vi "Request Refnum Release.vi"(8 "error in":errorcluster) -> (0 "error out":errorcluster)   [LabVIEW 2020, in "SECS Scenarios.lvlib" / "Scenarios Class.lvclass"]
uses:
  Scenarios Class.lvclass
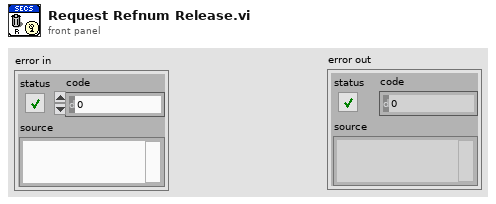
[diagram p1: front panel]
types:
  T1 = typedef "SECS Scenarios.lvlib/Scenarios Class.lvclass/Request Refnum.ctl" = cluster{"11-Alarm Management":refnum<user-event>, "07-Event Report From Equipment":refnum<user-event>, "14-Process Program Creating Editing or Deleting":refnum<user-event>, "21-Material Movement":refnum<user-event>, "23-Equipment Sends Information to Host":refnum<user-event>, "24-Host Accepts On-Line Request from Equipment":refnum<user-event>, "25-Host Refuses On-Line Request":refnum<user-event>, "29-Equipment Requests Time Value from Host":refnum<user-event>, "33-Update Trace Data":refnum<user-event>}
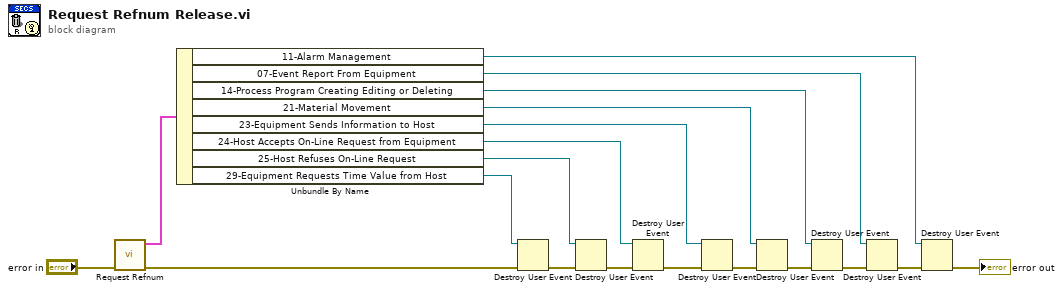
[diagram p0: block diagram]
diagram:
  n1 = call "Request Refnum.vi"("error in"="error in") -> ("error out"=w1:errorcluster, "Request Refnum"=w17:T1)  [unwired: 9 in]
  n2 = Unbundle By Name(w17) -> ("11-Alarm Management"=w8:refnum<user-event>, "07-Event Report From Equipment"=w9:refnum<user-event>, "14-Process Program Creating Editing or Deleting"=w10:refnum<user-event>, "21-Material Movement"=w11:refnum<user-event>, "23-Equipment Sends Information to Host"=w12:refnum<user-event>, "24-Host Accepts On-Line Request from Equipment"=w7:refnum<user-event>, "25-Host Refuses On-Line Request"=w4:refnum<user-event>, "29-Equipment Requests Time Value from Host"=w2:refnum<user-event>)
  n3 = Destroy User Event(user event=w2, error in=w1) -> (error out=w3:errorcluster)
  n4 = Destroy User Event(user event=w4, error in=w3) -> (error out=w5:errorcluster)
  n5 = Destroy User Event(user event=w7, error in=w5) -> (error out=w6:errorcluster)
  n6 = Destroy User Event(user event=w12, error in=w6) -> (error out=w15:errorcluster)
  n7 = Destroy User Event(user event=w11, error in=w15) -> (error out=w14:errorcluster)
  n8 = Destroy User Event(user event=w10, error in=w14) -> (error out=w13:errorcluster)
  n9 = Destroy User Event(user event=w9, error in=w13) -> (error out=w16:errorcluster)
  n10 = Destroy User Event(user event=w8, error in=w16) -> (error out=→"error out":errorcluster)
